vi "_028.vi"() -> ()   [LabVIEW 2024]
panel:
  out "error out":errorcluster
  # "Error Cluster :"
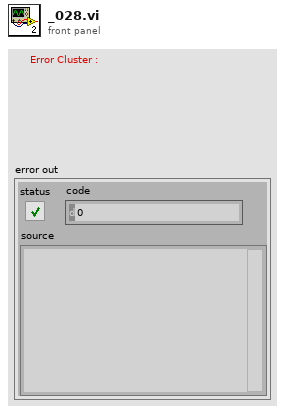
[diagram p1: front panel]
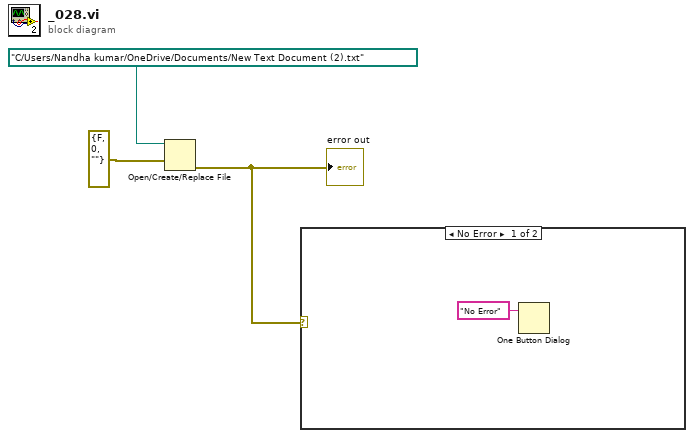
[diagram p0: block diagram]
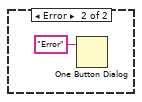
[diagram p2: hidden frame]
diagram:
  n1 = Open/Create/Replace File(file path (use dialog)=path "C:/Users/Nandha kumar/OneDrive/Documents/New Text Document (2).txt", error in=errorcluster {"status"=FALSE, "code"=0, "source"=""} ("error constant")) -> (error out=w2:errorcluster)  [unwired: 4 in, 2 out]
  "error out" <- w2
  n2 = case shown="No Error" w2 {
    frame No Error {
      n3 = One Button Dialog(message="No Error") -> ()  [unwired: 1 in, 1 out]
    }
    frame Error {
      n4 = One Button Dialog(message="Error") -> ()  [unwired: 1 in, 1 out]
    }
  }
